vi "Main.vi"() -> ()   [LabVIEW 2019]
doc: "The myRIO Project template acquires acceleration data from the onboard accelerometer and displays the changes of acceleration values in a waveform chart."
uses:
  <vilib>/myRIO/Instrument Drivers/Utilities/Utilities.lvlib
  <vilib>/myRIO/Express VI/Onboard IO/PWM/PWM Express VI.xnode
  <vilib>/myRIO/Instrument Drivers/Onboard IO/PWM/vis/Set Duty Cycle and Frequency.vi
  <vilib>/myRIO/Instrument Drivers/Onboard IO/PWM/PWM.lvlib
  <vilib>/myRIO/Instrument Drivers/Onboard IO/PWM/typedefs/PWM Configuration.ctl
  <vilib>/myRIO/Common/Instrument Driver Framework/myRIO v1.0/PWM/typedefs/PWM Channels Enum.ctl
  <vilib>/myRIO/Common/Instrument Driver Framework/Utilities/typedefs/Generic FPGA Reference.ctl
  <vilib>/myRIO/Common/Instrument Driver Framework/Utilities/typedefs/myRIO v1.0 Reference.ctl
  <vilib>/myRIO/Common/Instrument Driver Framework/Utilities/typedefs/Hardware Version Enum.ctl
  <vilib>/myRIO/Common/Instrument Driver Framework/Utilities/typedefs/myRIO Generic Hardware Reference.ctl
  <vilib>/myRIO/Instrument Drivers/Onboard IO/PWM/typedefs/PWM Reference.ctl
  <vilib>/myRIO/Instrument Drivers/Onboard IO/PWM/vis/myRIO PWM Open.xnode
  <vilib>/myRIO/Common/Instrument Driver Framework/Utilities/vis/Is FPGA Ref Available.vi
  <vilib>/myRIO/Common/Instrument Driver Framework/myRIO v1.0/PWM/vis/myRIO v1.1 Open PWM.vi
  <vilib>/userDefined/High Color/nirio_resource_hc.ctl
panel:
  out "error out 2":errorcluster
  in  "Rechtdoor?":bool
  in  "Rechts?":bool
  out "error out":errorcluster
  in  "Stop":bool
  # "Overview: The myRIO Project template acquires acceleration data from the onboard accelerometer and displays the changes of acceleration values in a waveform chart.\nInstructions:\n1. Check the myRIO target IP address in the project and make sure the target IP address is correct. \n2. Run this VI."
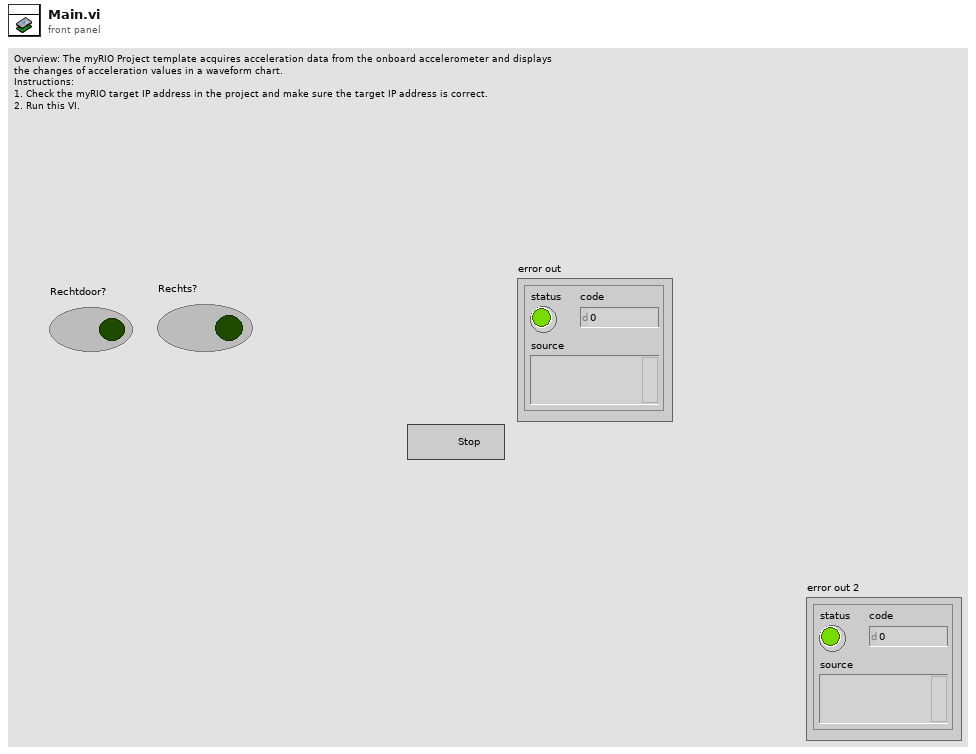
[diagram p1: front panel]
types:
  T1 = typedef "PWM.lvlib/PWM Reference.ctl" = cluster{"myRIO Reference":T2, "PWM Channels Enum":T6, "PWM Configuration":T7}
  T2 = typedef "myRIO Generic Hardware Reference.ctl" = cluster{"myRIO Model":T3, "myRIO Hardware Reference":T4}
  T3 = typedef "Hardware Version Enum.ctl" = enum16{"Unknown", "myRIO-1900", "myRIO-1950", "roboRIO", "NI ELVIS RIO CM", "ELVIS III"}
  T4 = typedef "myRIO v1.0 Reference.ctl" = cluster{"Generic FPGA Reference":T5, "Allow multiple opens":bool}
  T5 = typedef "Generic FPGA Reference.ctl" = refnum<k20>
  T6 = typedef "PWM Channels Enum.ctl" = enum16{"Not Connected", "C/PWM0", "C/PWM1", "A/PWM0", "A/PWM1", "A/PWM2", "A/PWM3", "A/PWM4", "A/PWM5", "A/PWM6", "A/PWM7", "A/PWM8", "A/PWM9", "A/PWM10", "A/PWM11", "A/PWM12", "A/PWM13", "A/PWM14", "A/PWM15", "A/PWM16", "A/PWM17", "A/PWM18", "A/PWM19", "B/PWM0", "B/PWM1", "B/PWM2", "B/PWM3", "B/PWM4", "B/PWM5", "B/PWM6", "B/PWM7", "B/PWM8", "B/PWM9", "B/PWM10", "B/PWM11", "B/PWM12", "B/PWM13", "B/PWM14", "B/PWM15", "B/PWM16", "B/PWM17", "B/PWM18", "B/PWM19", "PWM/PWM0", "PWM/PWM1", "PWM/PWM2", "PWM/PWM3", "PWM/PWM4", "PWM/PWM5", "PWM/PWM6", "PWM/PWM7", "PWM/PWM8", "PWM/PWM9"}
  T7 = typedef "PWM.lvlib/PWM Configuration.ctl" = cluster{"Frequency":dbl, "Duty Cycle":dbl}
  T8 = typedef "nirio_resource_hc.ctl" = tag
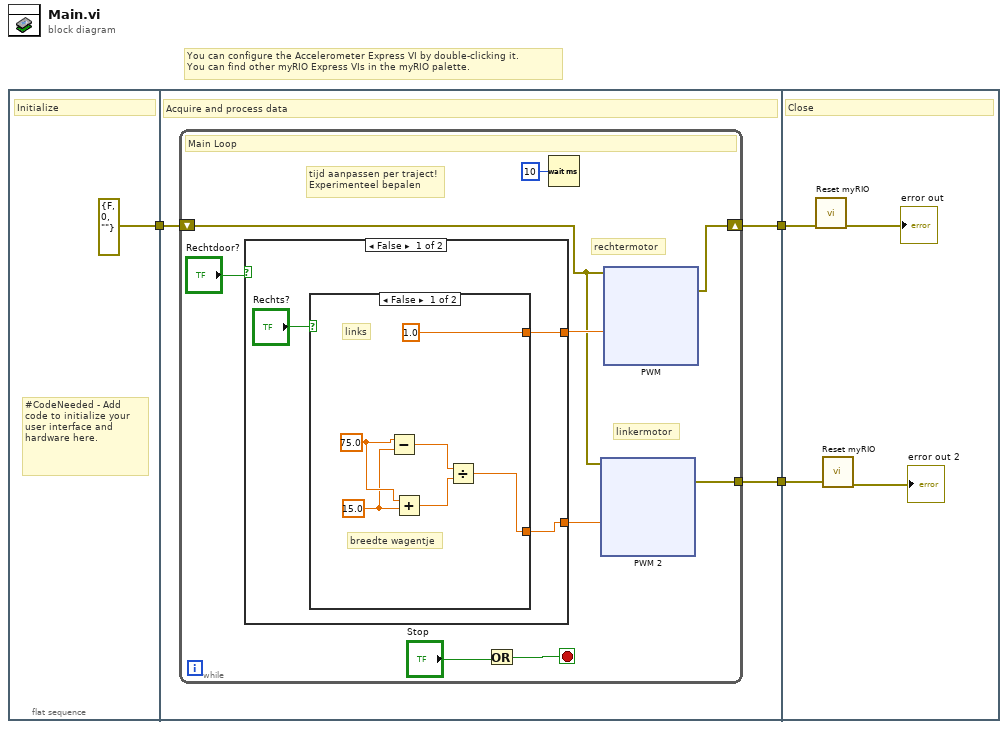
[diagram p0: block diagram]
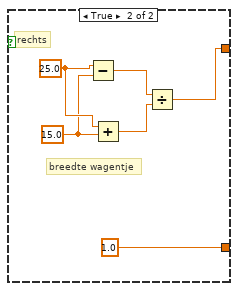
[diagram p2: hidden frame]
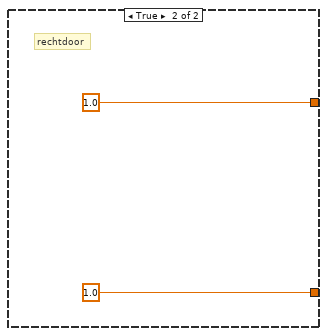
[diagram p3: hidden frame]
diagram:
  # "You can configure the Accelerometer Express VI by double-clicking it.\nYou can find other myRIO Express VIs in the myRIO palette."
  n1 = flat-sequence {
    tunnel: [errorcluster {"status"=FALSE, "code"=0, "source"=""} ("error in (no error)")] -> w3
    tunnel: w3 -> [w7]
    tunnel: [w6] -> w2
    tunnel: [w5] -> w1
    tunnel: w2 -> [w104]
    tunnel: w1 -> [w106]
    frame #0 {
      # "#CodeNeeded - Add code to initialize your user interface and hardware here."
      # "Initialize"
    }
    frame #1 {
      # "Acquire and process data"
      n2 = while {
        shift-right: [w9] -> w5
        shift-left: w7 -> [w10]
        tunnel: [w8] -> w6
        stop <- w15 stop-if-true
        # "tijd aanpassen per traject!\nExperimenteel bepalen"
        # "linkermotor"
        # "rechtermotor"
        # "Main Loop"
        n3 = case shown="False" "Rechtdoor?" {
          tunnel: [w18 1.0] -> w11
          tunnel: [w17 1.0] -> w12
          frame False {
            n4 = case shown="False" "Rechts?" {
              tunnel: [1.0 w26] -> w18
              tunnel: [w20 1.0] -> w17
              frame False {
                w23 = 15.0
                w24 = 75.0
                # "breedte wagentje"
                # "links"
                n5 = Subtract(x=w24, y=w23) -> (x-y=w22:dbl)
                n6 = Add(x=w24, y=w23) -> (x+y=w21:dbl)
                n7 = Divide(x=w22, y=w21) -> (x/y=w20:dbl)
              }
              frame True {
                w29 = 15.0
                w30 = 25.0
                # "breedte wagentje"
                # "rechts"
                n8 = Subtract(x=w30, y=w29) -> (x-y=w28:dbl)
                n9 = Add(x=w30, y=w29) -> (x+y=w27:dbl)
                n10 = Divide(x=w28, y=w27) -> (x/y=w26:dbl)
              }
            }
          }
          frame True {
            # "rechtdoor"
          }
        }
        n11 = Or(y="Stop") -> (x .or. y?=w15:bool)  [unwired: 1 in]
        n12 = Wait (ms)(milliseconds to wait=u32 10) -> ()  [unwired: 1 out]
        n13 = xnode "PWM 2"("Duty Cycle"=w12, "error in (no error)"=w10) -> ("error out"=w8:errorcluster)  [unwired: 1 in]
        n14 = xnode "PWM"("Duty Cycle"=w11, "error in (no error)"=w10) -> ("error out"=w9:errorcluster)  [unwired: 1 in]
      }
    }
    frame #2 {
      # "Close"
      n15 = call <vilib>:"Reset myRIO.vi"("error in (no error)"=w106) -> ("error out"=→"error out":errorcluster)  [unwired: 10 in]
      n16 = call <vilib>:"Reset myRIO.vi"("error in (no error)"=w104) -> ("error out"=→"error out 2":errorcluster)  [unwired: 10 in]
    }
  }
